vi "Reset Layer VI.vi"(8 "error in (no error)":errorcluster) -> (0 "error out":errorcluster)   [LabVIEW 2021]
uses:
  vi.lib/LabVIEW Icon API/lv_icon/lv_icon.lvlib
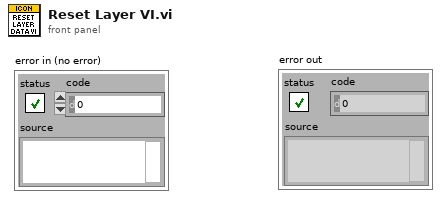
[diagram p1: front panel]
types:
  T1 = typedef "Who Invoked Icon Editor.ctl" = cluster{"Icon Editor Invoker Type":T2, "App Refnum of Invoker":refnum<vi>, "Qualified Name of Invoker":string, "Path to Invoker":path}
  T2 = typedef "Icon Editor Invoker Type.ctl" = enum32{"Unknown Icon Source", "VI Icon", "Library Icon (any library type)", "Palette icon", "Icon from App Method"}
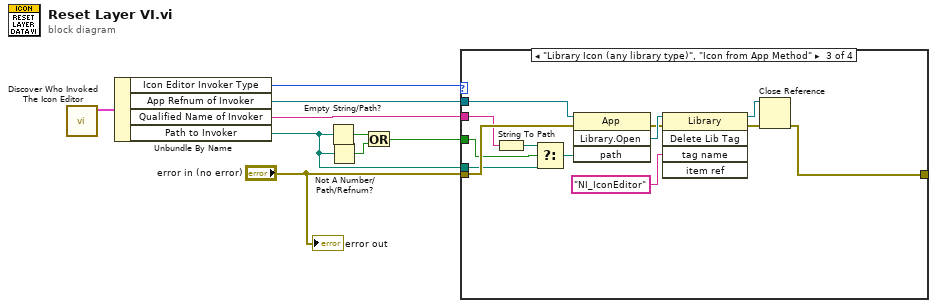
[diagram p0: block diagram]
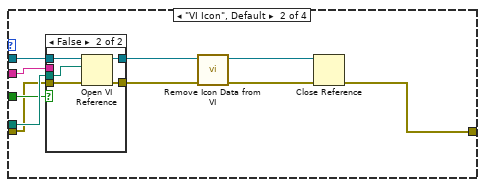
[diagram p3: hidden frame]
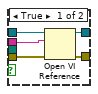
[diagram p4: hidden frame]
diagram:
  n1 = call <resource>:"Discover Who Invoked The Icon Editor.vi"() -> ("Who Invoked The Icon Editor?"=w9:T1)  [unwired: 11 out]
  n2 = Unbundle By Name(w9) -> ("Icon Editor Invoker Type"=w6:T2, "App Refnum of Invoker"=w7:refnum<vi>, "Qualified Name of Invoker"=w8:string, "Path to Invoker"=w1:path)
  n3 = Empty String/Path?(string/path=w1) -> (empty?=w4:bool)
  n4 = Not A Number/Path/Refnum?(number/path/refnum=w1) -> (NaN/Path/Refnum?=w3:bool)
  n5 = Or(x=w4, y=w3) -> (x .or. y?=w2:bool)
  n6 = case shown="\"Library Icon (any library type)\", \"Icon from App Method\"" w6 {
    tunnel: "error in (no error)" -> [w10 w15 w37 w44]
    tunnel: [w10 w20 w42 w44] -> _
    tunnel: w8 -> [_ w18 w35 _]
    tunnel: w7 -> [_ w19 w43 _]
    tunnel: w2 -> [_ w16 w34 _]
    tunnel: w1 -> [_ w17 w33 _]
    frame "Unknown Icon Source" {
    }
    frame "VI Icon", Default {
      n7 = case shown="False" w16 {
        tunnel: w15 -> [w25 w30]
        tunnel: [w24 w29] -> w14
        tunnel: [w23 w28] -> w13
        tunnel: w19 -> [w22 w27]
        tunnel: w18 -> [w21 _]
        tunnel: w17 -> [_ w26]
        frame True {
          n8 = Open VI Reference(application reference (local)=w22, vi path=w21, error in (no error)=w25) -> (vi reference=w24:refnum<vi>, error out=w23:errorcluster)  [unwired: 3 out]
        }
        frame False {
          n9 = Open VI Reference(application reference (local)=w27, vi path=w26, error in (no error)=w30) -> (vi reference=w29:refnum<vi>, error out=w28:errorcluster)  [unwired: 3 out]
        }
      }
      n10 = call "Remove Icon Data from VI.vi"("error in (no error)"=w13, "VI Ref in"=w14) -> ("error out"=w12:errorcluster, "VI Ref out"=w11:refnum<vi>)  [unwired: 8 in]
      n11 = Close Reference(reference=w11, error in (no error)=w12) -> (error out=w20:errorcluster)
    }
    frame "Library Icon (any library type)", "Icon from App Method" {
      n12 = String To Path(string=w35) -> (path=w36:path)
      n13 = Select(t=w36, s=w34, f=w33) -> (s? t:f=w32:path)
      n14 = invoke class="App" method="Library.Open"(reference=w43, error in=w37, "path"=w32) -> (error out=w40:errorcluster, "Open Library"=w41:refnum<vi>)  [unwired: 1 in, 2 out]
      n15 = invoke class="Library" method="Delete Lib Tag"(reference=w41, error in=w40, "tag name"="NI_IconEditor" ("Tag Name")) -> (reference out=w38:refnum<vi>, error out=w39:errorcluster)  [unwired: 2 in, 3 out]
      n16 = Close Reference(reference=w38, error in (no error)=w39) -> (error out=w42:errorcluster)
    }
    frame "Palette icon" {
    }
  }
  "error out" <- "error in (no error)"
